vi "Init Active Devices.vi"(8 "error in":errorcluster, 10 "Device Names":string, 11 "DAC CS Humid in":refnum<class "DAC CS Humid.lvclass">) -> (0 "error out":errorcluster, 3 "DAC CS Humid out":refnum<class "DAC CS Humid.lvclass">)   [LabVIEW 2019, in "DAC.lvlib" / "DAC CS Humid.lvclass"]
uses:
  DAC CS Humid.lvclass
  C:/Users/krio/Documents/LV_Projects/test-stand/App/DAC/DAC.lvclass
  DAC.lvclass/DAC.ctl
  DAC CS Humid.lvclass/DAC CS Humid.ctl
  DAC.lvclass
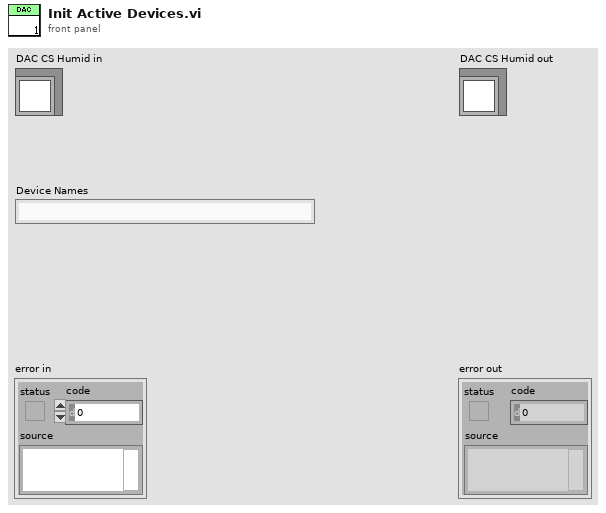
[diagram p1: front panel]
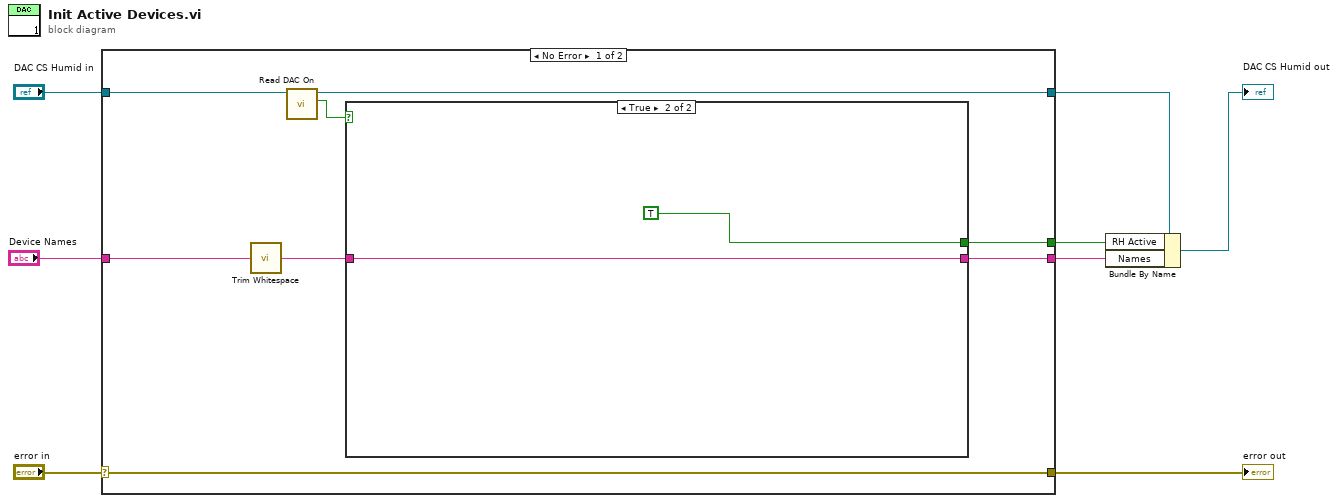
[diagram p0: block diagram]
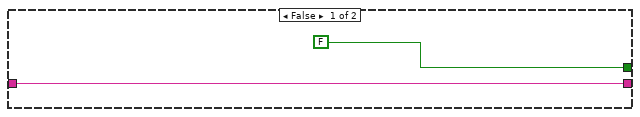
[diagram p2: hidden frame]
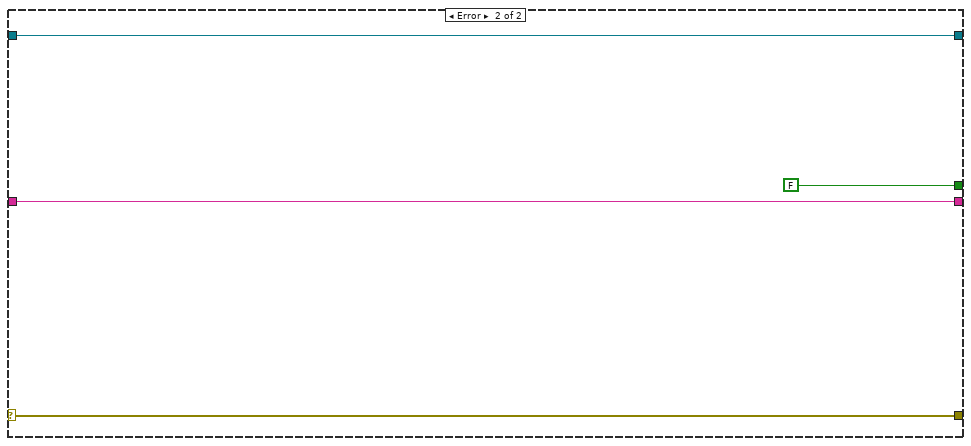
[diagram p3: hidden frame]
diagram:
  n1 = case shown="No Error" "error in" {
    selector: "error in" -> [w16 w24]
    tunnel: [w16 w24] -> w7
    tunnel: [w14 w23] -> w5
    tunnel: "DAC CS Humid in" -> [w15 w23]
    tunnel: "Device Names" -> [w12 w21]
    tunnel: [w10 w21] -> w2
    tunnel: [w9 FALSE] -> w1
    frame No Error {
      n2 = call <vilib>:"Trim Whitespace.vi"("string"=w12) -> ("trimmed string"=w11:string)  [unwired: 1 in]
      n3 = call "Read DAC On.vi"("DAC in"=w15) -> ("DAC On"=w13:bool, "DAC out"=w14:refnum<class "DAC CS Humid.lvclass">)  [unwired: 8 in, 1 out]
      n4 = case shown="True" w13 {
        tunnel: w11 -> [w17 w20]
        tunnel: [w17 w20] -> w10
        tunnel: [FALSE TRUE] -> w9
        frame False {
        }
        frame True {
        }
      }
    }
    frame Error {
    }
  }
  "error out" <- w7
  n5 = Bundle By Name(cluster=w5, "RH Active"=w1, "Names"=w2) -> (→"DAC CS Humid out":refnum<class "DAC CS Humid.lvclass">)
